vi "Ok to proceed check.vi"() -> (0 "Error":errorcluster, 1 "DLL version":string)   [LabVIEW 2014]
uses:
  Laser enum.ctl
  Commands.ctl
  Coherent global.vi
panel:
  # "PN 05/11/2014"
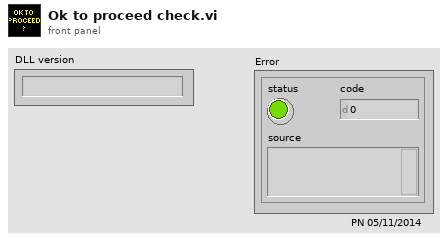
[diagram p1: front panel]
types:
  T1 = typedef "Commands.ctl" = u8
  T2 = typedef "Laser enum.ctl" = u8
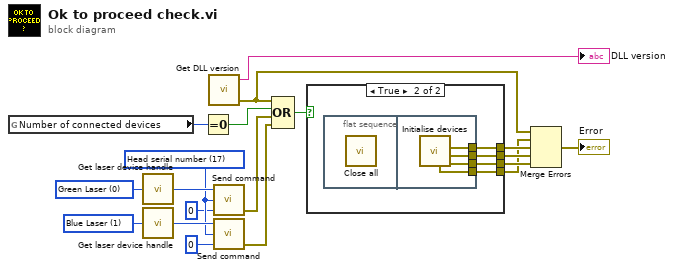
[diagram p0: block diagram]
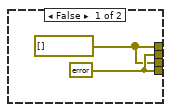
[diagram p2: hidden frame]
diagram:
  w11 = T1 17 items=["Measured main TEC temperature"=0, "Measured SHG heater temperature"=1, "Measured BRF heater temperature"=2, "Main TEC temperature command"=3, "SHG heater temperature command"=4, "BRF heater temperature command"=5, "Main TEC drive"=6, "SHG heater drive"=7, "BRF heater drive"=8, "Output power from photodiode"=9, "Output power setpoint (Get)"=10, "Output power setpoint (Set)"=11, "Start-up power setting (Get)"=12, "Start-up power setting (Set)"=13, "Measured LDD current"=14, "Maximum LDD current limit"=15, "16-bit fault code"=16, "Head serial number"=17, "Head board rev"=18, "Head type"=19, "LDD enable state"=20, "Key switch command (Get)"=24, "Key switch command (Set)"=25, "Key switch actual"=26, "Interlock status"=27, "Head hours"=28, "Photo or current mode command (Get)"=29, "Photo or current mode command (Set)"=30, "Photo or current mode actual"=31, "Analog input enable command (Get)"=32, "Analog input enable command (Set)"=33, "Analog input actual"=34, "Power supply glue input"=36, "Power supply glue output"=37] ("Command")
  w14 = T2 1 items=["Green Laser", "Blue Laser"] ("Selected laser")
  w15 = T2 0 items=["Green Laser", "Blue Laser"] ("Selected laser")
  n1 = global read "Coherent global.vi" "Number of connected devices"() -> (w19:u32)
  n2 = call "Get laser device handle.vi"("Selected laser"=w15) -> ("Device handle"=w13:u32)
  n3 = call "Get laser device handle.vi"("Selected laser"=w14) -> ("Device handle"=w12:u32)
  n4 = Equal To 0?(x=w19) -> (x = 0?=w18:bool)
  n5 = call "Get DLL version.vi"() -> ("Error"=w3:errorcluster, "DLL version"=→"DLL version":string)  [unwired: 1 in]
  n6 = call "Send command.vi"("Value"=u16 0, "Command"=w11, "Device handle"=w13) -> ("Error"=w8:errorcluster)  [unwired: 2 out]
  n7 = call "Send command.vi"("Value"=u16 0, "Command"=w11, "Device handle"=w12) -> ("Error"=w7:errorcluster)  [unwired: 2 out]
  n8 = Compound Arithmetic op=OR(w3, w18, w8, w7) -> (w17:bool)
  n9 = case shown="True" w17 {
    tunnel: [w20 w25] -> w6
    tunnel: [w21 w24] -> w5
    tunnel: [w20 w23] -> w4
    tunnel: [w21 w22] -> w2
    frame False {
      w21 = errorcluster {"status"=FALSE, "code"=0, "source"=""} ("Device detection error")
      w20 = errorcluster[] [] ("Device initialisation errors")
    }
    frame True {
      n10 = flat-sequence {
        tunnel: [w29] -> w25
        tunnel: [w28] -> w24
        tunnel: [w27] -> w23
        tunnel: [w26] -> w22
        frame #0 {
          n11 = call "Close all.vi"() -> ()  [unwired: 1 out]
        }
        frame #1 {
          n12 = call "Initialise devices.vi"() -> ("Laser comms. error"=w29:errorcluster[], "Get lasers serial num. error"=w26:errorcluster, "Device detection error"=w28:errorcluster, "Device initialisation errors"=w27:errorcluster[])  [unwired: 5 in, 2 out]
        }
      }
    }
  }
  n13 = Merge Errors(w3, w2, w6, w5, w4) -> (→"Error":errorcluster)
